vi "SelectChannels.vi"(6 "Controls Only?":bool, 8 "error in":errorcluster, 9 "Listbox Settings":T1, 10 "Previous Selection":T2[](array[typedef]), 11 "Root.BaseNodeType":refnum<k24>) -> (0 "error out":errorcluster, 1 "Listbox Settings Out":T1, 2 "Channel Selection":T2[](array[typedef]))   [LabVIEW 2012, in "TableSupportLib.lvlib"]
uses:
  TableSupportLib.lvlib
  NationalInstruments.VeriStand.SystemStorageUI
  Table_ChannelInfoCluster.ctl
  NationalInstruments.VeriStand.SystemStorage
  Table_ListboxSettings.ctl
  <vilib>/Utility/miscctls.llb/LVRowAndColumnTypeDef.ctl
  <vilib>/Utility/miscctls.llb/LVRowAndColumnUnsignedTypeDef.ctl
  <vilib>/NI Veristand/UI Controls/Tree and Alias Browser/Node Ref.ctl
  NationalInstruments.VeriStand
  <vilib>/NI/AMC/Read Termination Message.vi
  <vilib>/NI/AMC/Create Single Message.vi
  <vilib>/NI/AMC/Update Message Routing Info.vi
  Table_Globals.vi
  <vilib>/NI/AMC/Globals.vi
  <vilib>/NI/AMC/Send Message.vi
  NationalInstruments.VeriStand.SystemDefinitionAPI
  <vilib>/NI/AMC/AMC.lvlib
  <vilib>/NI Veristand/UI Controls/Tree and Alias Browser/NI_VS UI Tree Alias Browser.lvlib
panel:
  in  "Tab Control":enum32{"Channel Setup", "Listbox Setup"}(tab)
  in  "Select Channels":refnum<k24>(container)
  in  "Channels":i32[](listbox)
  in  "Remove":bool
  in  "Add":bool
  in  "Generate Template":bool
  in  "Path":path
  in  "Include Limits":bool
  in  "Poll Rate":u32(ring)=200 items=["15 Hz"=66, "10 Hz"=100, "5 Hz"=200, "1 Hz"=1000, ".5"=2000]
  in  "Bold":bool
  in  "Text Size":u32=13
  in  "Cancel":bool
  in  "OK":bool
  # "Rate"
  # "Limits"
  # "Text"
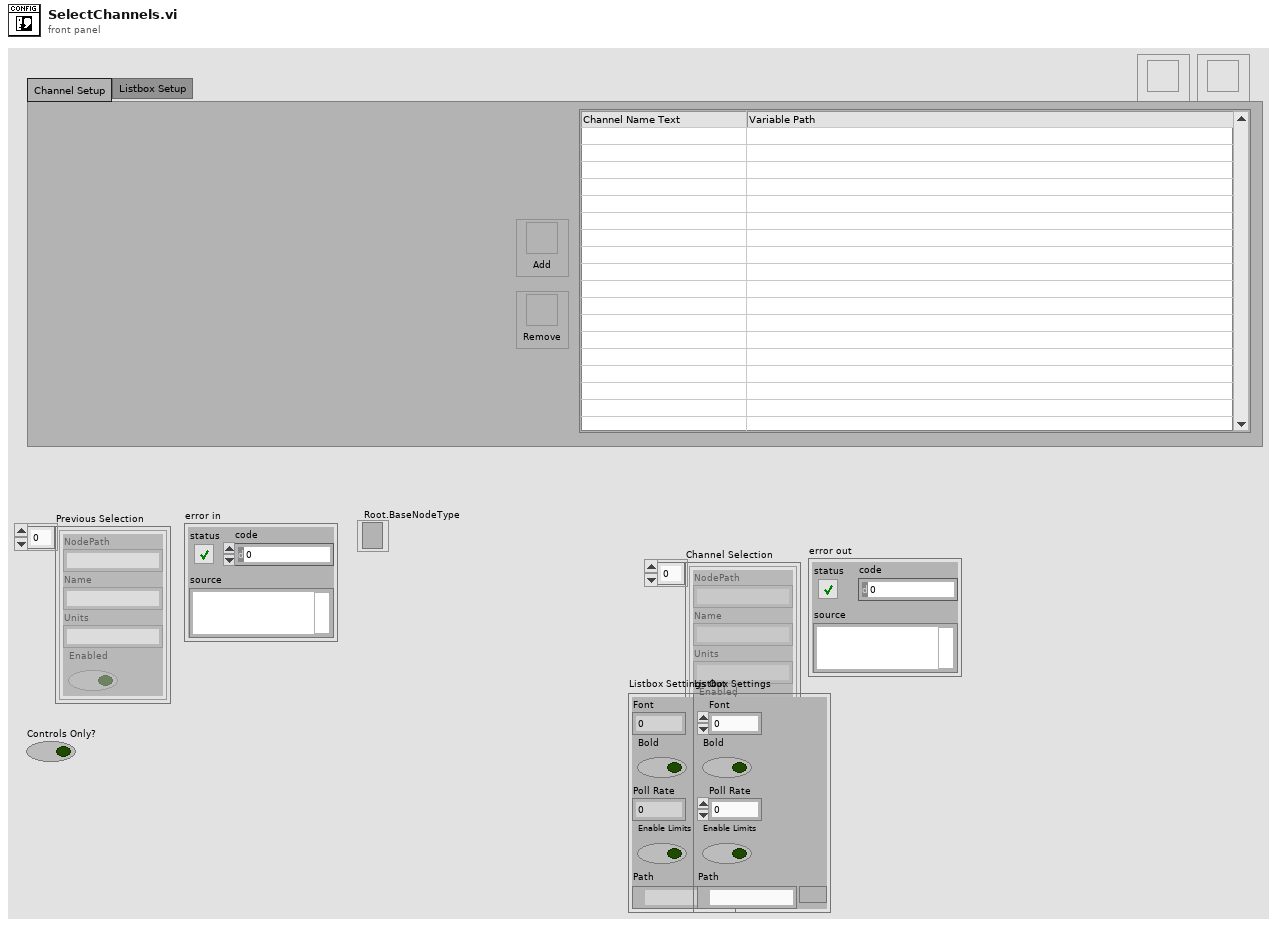
[diagram p1: front panel]
types:
  T1 = typedef "TableSupportLib.lvlib/Table_ListboxSettings.ctl" = cluster{"Font":u32, "Bold":bool, "Poll Rate":u32, "Enable Limits":bool, "Path":path}
  T2 = typedef "TableSupportLib.lvlib/Table_ChannelInfoCluster.ctl" = cluster{"NodePath":string, "Name":string, "Units":string, "Enabled":bool}
  T3 = typedef "NI_VS UI Tree Alias Browser.lvlib/Callback Type.ctl" = cluster{"Net Callbacks":refnum<k27>[], "Event":T4}
  T4 = typedef "NI_VS UI Tree Alias Browser.lvlib/Net Event Data Ref.ctl" = refnum<user-event>
  T5 = typedef "NI_VS UI Tree Alias Browser.lvlib/Tree Alias Browser Ref.ctl" = refnum<k24>
  T6 = typedef "AMC.lvlib/Message Queue.ctl" = refnum<queue>
  T7 = typedef "NI_VS UI Tree Alias Browser.lvlib/Node Ref.ctl" = refnum<k24>
  T8 = typedef "LVRowAndColumnUnsignedTypeDef.ctl" = cluster{"Row":u32, "Column":u32}
  T9 = typedef "LVRowAndColumnTypeDef.ctl" = cluster{"Row":i32, "Column":i32}
  T10 = enum16{"open", "replace", "create", "open or create", "replace or create", "replace or create with confirmation"}
  T11 = typedef "NI_VS UI Tree Alias Browser.lvlib/Net Event.ctl" = enum16{"SelectedItem", "DblClick"}
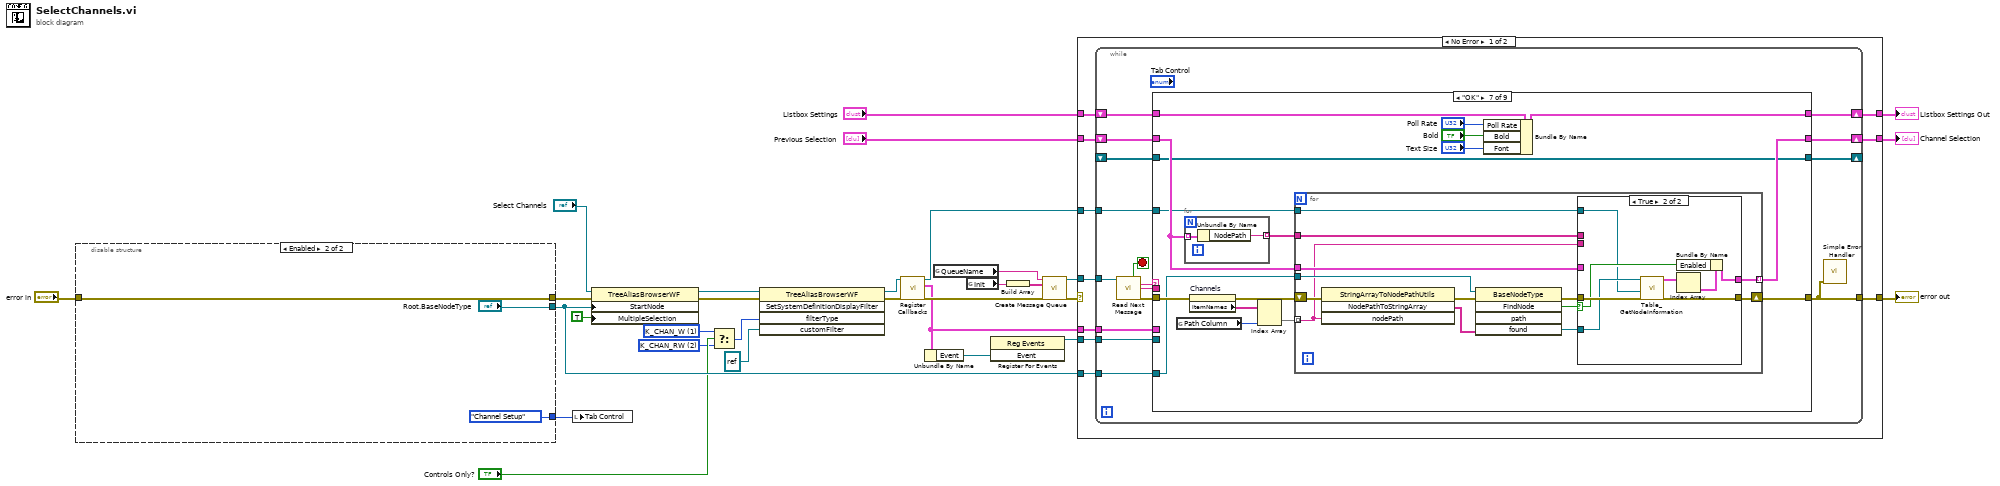
[diagram p0: block diagram]
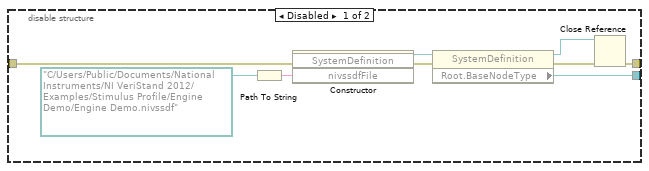
[diagram p2: hidden frame]
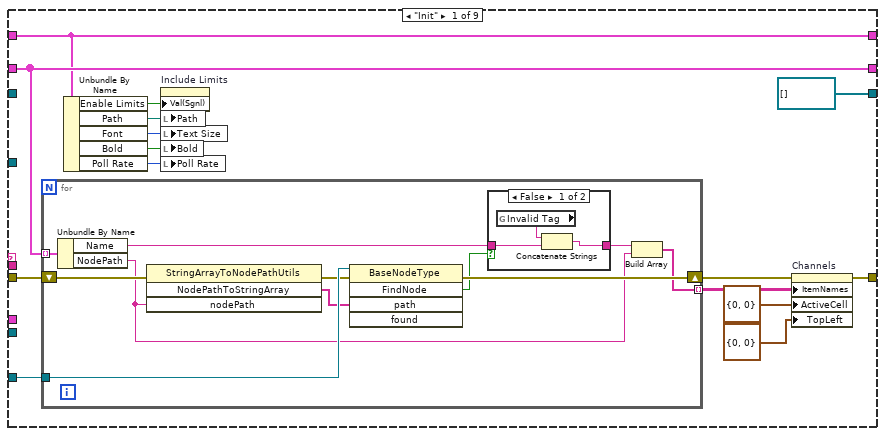
[diagram p3: hidden frame]
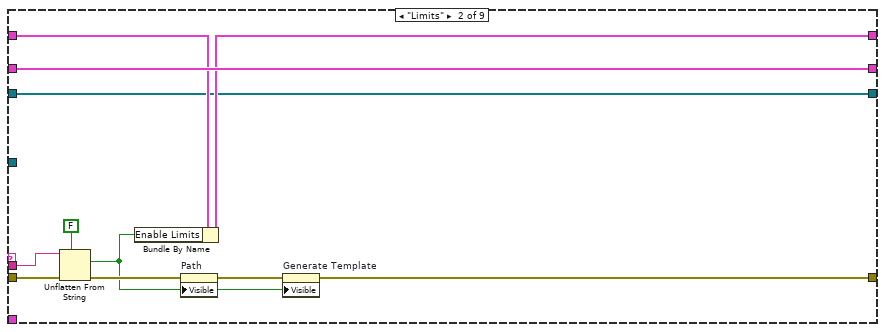
[diagram p5: hidden frame]
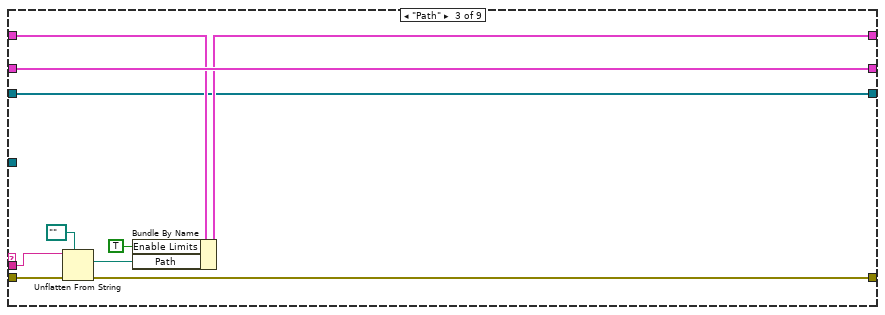
[diagram p6: hidden frame]
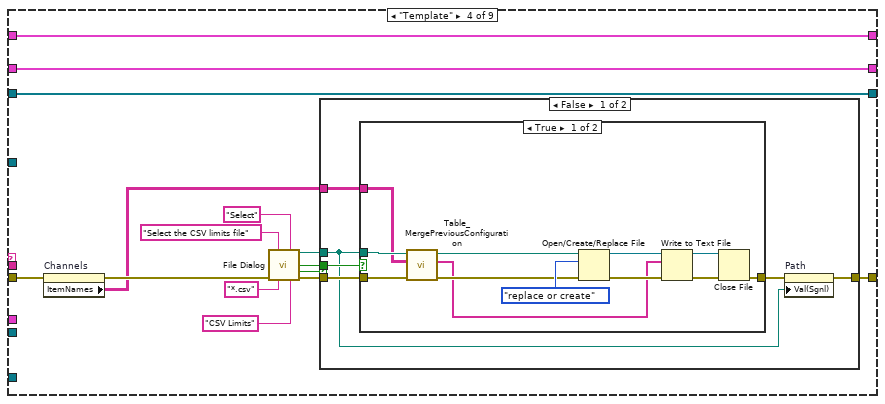
[diagram p7: hidden frame]
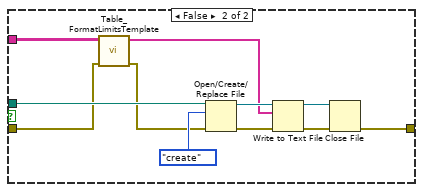
[diagram p8: hidden frame]
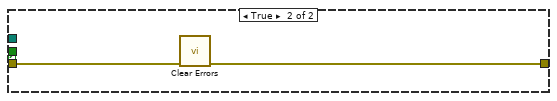
[diagram p9: hidden frame]
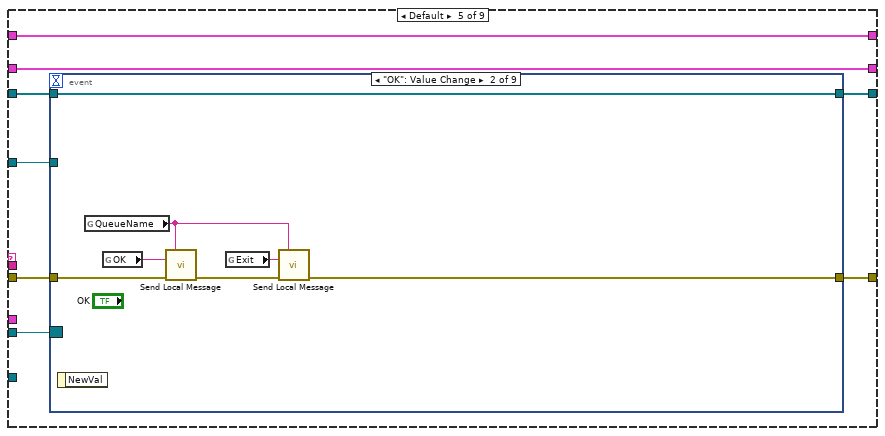
[diagram p10: hidden frame]
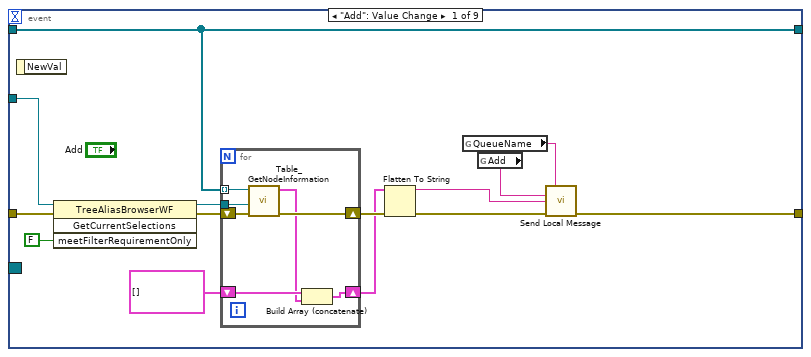
[diagram p11: hidden frame]
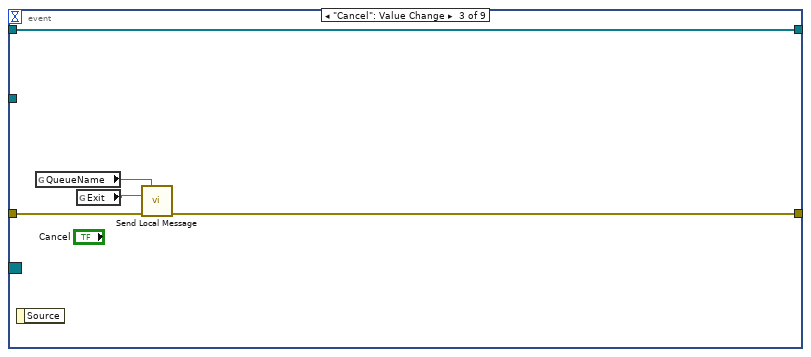
[diagram p12: hidden frame]
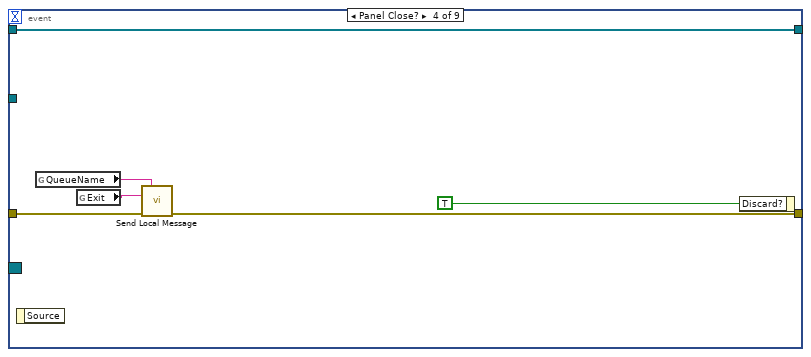
[diagram p13: hidden frame]
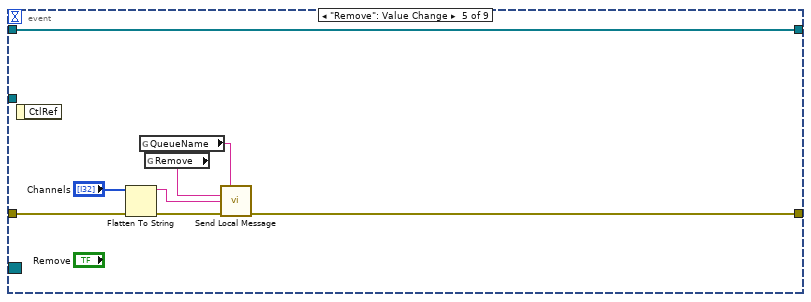
[diagram p14: hidden frame]
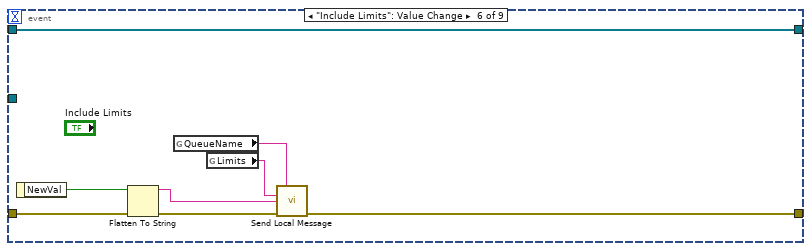
[diagram p15: hidden frame]
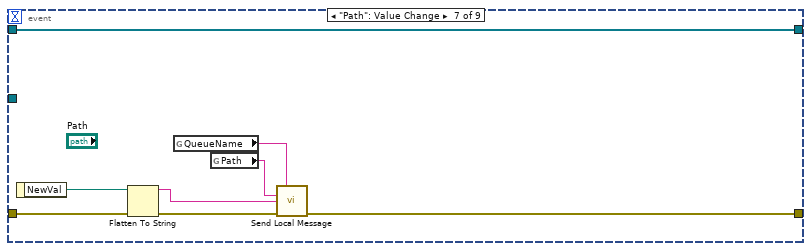
[diagram p16: hidden frame]
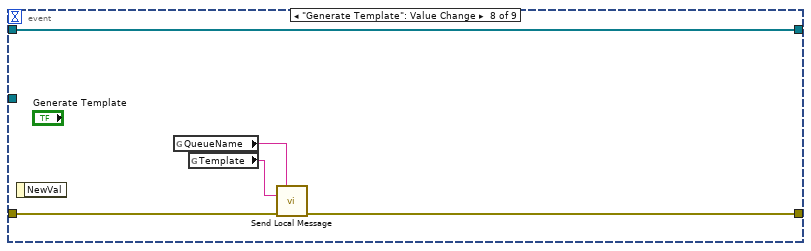
[diagram p17: hidden frame]
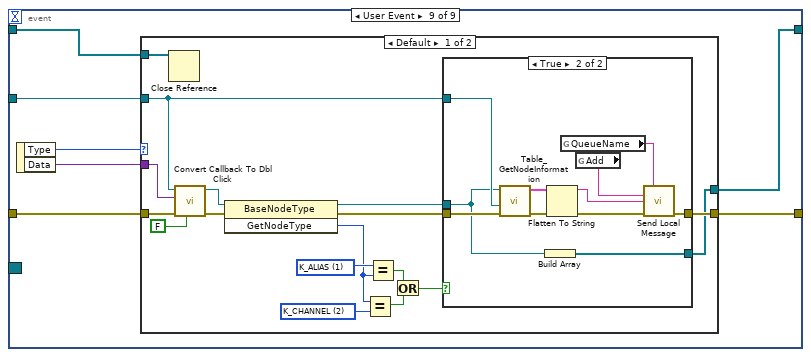
[diagram p18: hidden frame]
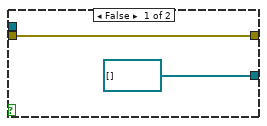
[diagram p19: hidden frame]
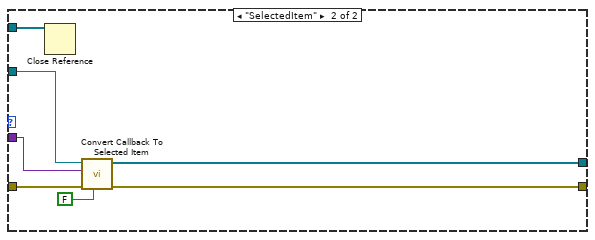
[diagram p20: hidden frame]
diagram:
  w9 = u8 1 items=["K_CHAN_R", "K_CHAN_W", "K_CHAN_RW", "K_CHAN_VOLT", "K_CHAN_FAULT", "K_ALL", "K_CUSTOM", "K_CHAN_R_VIS", "K_CHAN_W_VIS", "K_CHAN_RW_VIS", "K_CHAN_VOLT_VIS", "K_CHAN_FAULT_VIS", "K_WAVE", "K_WAVE_VIS", "K_WAVE_DBL", "K_WAVE_CDB", "K_WAVE_DBL_VIS", "K_WAVE_CDB_VIS"] ("filterType")
  w10 = u8 2 items=["K_CHAN_R", "K_CHAN_W", "K_CHAN_RW", "K_CHAN_VOLT", "K_CHAN_FAULT", "K_ALL", "K_CUSTOM", "K_CHAN_R_VIS", "K_CHAN_W_VIS", "K_CHAN_RW_VIS", "K_CHAN_VOLT_VIS", "K_CHAN_FAULT_VIS", "K_WAVE", "K_WAVE_VIS", "K_WAVE_DBL", "K_WAVE_CDB", "K_WAVE_DBL_VIS", "K_WAVE_CDB_VIS"] ("filterType")
  n1 = disable-structure shown="Enabled" {
    disable-tunnel: [w35 "Root.BaseNodeType"] -> w23
    disable-tunnel: [w32 w42] -> w19
    disable-tunnel: "error in" -> [w31 w42]
    disable-tunnel: [_ enum32{"Channel Setup", "Listbox Setup"}."Channel Setup" ("Tab Control")] -> w12
    frame Disabled {
      n2 = Path To String(path=path "C:/Users/Public/Documents/National Instruments/NI VeriStand 2012/Examples/Stimulus Profile/Engine Demo/Engine Demo.nivssdf") -> (string=w38:string)
      n3 = constructor class="SystemDefinition"(error in=w31, "nivssdfFile"=w38) -> (reference out=w37:refnum<k24>, error out=w36:errorcluster)  [unwired: 2 in, 2 out]
      n4 = property class="SystemDefinition"(reference=w37, error in=w36) -> (reference out=w34:refnum<k24>, error out=w33:errorcluster, "Root.BaseNodeType"=w35:refnum<k24>)
      n5 = Close Reference(reference=w34, error in (no error)=w33) -> (error out=w32:errorcluster)
    }
    frame Enabled {
    }
  }
  n6 = local write "Tab Control"(w12) -> ()
  n7 = property class="TreeAliasBrowserWF"(reference="Select Channels", error in=w19, "StartNode"=w23, "MultipleSelection"=TRUE) -> (reference out=w29:refnum<k24>, error out=w28:errorcluster)
  n8 = Select(t=w9, s="Controls Only?", f=w10) -> (s? t:f=w8:u8)
  n9 = invoke class="TreeAliasBrowserWF" method="SetSystemDefinitionDisplayFilter"(reference=w29, error in=w28, "filterType"=w8, "customFilter"=refnum<k24> refnum) -> (reference out=w5:refnum<k24>, error out=w7:errorcluster)  [unwired: 1 in, 3 out]
  n10 = call <vilib>:"Register Callbacks.vi"("error in (no error)"=w7, "Tree Alias"=w5) -> ("error out"=w6:errorcluster, "Callbacks"=w1:T3, "Tree Alias dup"=w4:T5)  [unwired: 7 in]
  n11 = Unbundle By Name(w1) -> ("Event"=w2:T4)
  n12 = global read "Table_Globals.vi" "QueueName"() -> (w25:string)
  n13 = global read "Table_Globals.vi" "Init"() -> (w21:string)
  n14 = register-events(w2) -> (reference out=w3:refnum<event-registration>)  [unwired: 2 in, 1 out]
  n15 = Build Array(w21) -> (w20:string[])
  n16 = call <vilib>:"Create Message Queue.vi"("message queue name"=w25, "initial message names"=w20, "error in"=w6) -> ("message queue out"=w26:T6, "error out"=w18:errorcluster)  [unwired: 11 in]
  n17 = case shown="No Error" w18 {
    selector: w18 -> [_ w401]
    tunnel: w4 -> [w52 _]
    tunnel: w26 -> [w51 _]
    tunnel: "Previous Selection" -> [w50 w402]
    tunnel: [w49 w400] -> w15
    tunnel: w23 -> [w48 _]
    tunnel: [w47 w402] -> w22
    tunnel: "Listbox Settings" -> [w46 w399]
    tunnel: [w45 w399] -> w13
    tunnel: w3 -> [w44 _]
    tunnel: w1 -> [w43 _]
    frame No Error {
      n18 = while {
        tunnel: w52 -> [w68]
        tunnel: w51 -> [w66]
        tunnel: [w59] -> w49
        tunnel: w48 -> [w62]
        shift-right: [w61] -> w47
        shift-left: w50 -> [w63]
        shift-right: [w57] -> w45
        shift-left: w46 -> [w58]
        tunnel: w44 -> [w56]
        shift-right: [w55] -> _
        shift-left: _ -> [w54]
        tunnel: w43 -> [w53]
        stop <- w60 stop-if-true
        n19 = call <vilib>:"Read Next Message.vi"("message queue in"=w66) -> ("exit process?"=w60:bool, "message name"=w65:string, "message value"=w64:string, "error out"=w67:errorcluster)  [unwired: 7 in, 4 out]
        n20 = case shown="\"OK\"" w65 {
          tunnel: w68 -> [_ _ _ _ w173 _ w318 w374 _]
          tunnel: w67 -> [w82 w108 w118 w132 w172 w298 w333 w368 w394]
          tunnel: [w79 w103 w117 w124 w171 w295 w329 w373 w383] -> w59
          tunnel: w64 -> [_ w107 w116 _ _ w297 _ _ w392]
          tunnel: w63 -> [w83 w109 w119 w134 w170 w296 w325 w377 w382]
          tunnel: w62 -> [w81 _ _ _ _ _ w331 _ _]
          tunnel: [w83 w109 w119 w134 w170 w296 w327 w377 w382] -> w61
          tunnel: [w72 w101 w112 w133 w169 w287 w319 w372 w379] -> w57
          tunnel: w58 -> [w72 w102 w113 w133 w169 w287 w320 w372 w379]
          tunnel: w56 -> [_ _ _ _ w168 _ _ w367 _]
          tunnel: [T7[] [] ("Selected Items") w99 w110 w120 w167 w286 w317 T7[] [] ("Selected Items") w378] -> w55
          tunnel: w54 -> [_ w99 w110 w120 w166 w286 w317 w371 w378]
          tunnel: w53 -> [_ _ _ _ _ _ _ w369 _]
          frame "Init" {
            n21 = for {
              tunnel: w81 -> [w94]
              shift-right: [w89] -> w80
              shift-left: w82 -> [w93]
              tunnel: w83 -> [w92] mode=indexing
              tunnel: [w87] -> w78 mode=indexing
              n22 = Unbundle By Name(w92) -> ("Name"=w86:string, "NodePath"=w84:string)
              n23 = invoke class="StringArrayToNodePathUtils" method="NodePathToStringArray"(error in=w93, "nodePath"=w84) -> (error out=w90:errorcluster, "NodePathToStringArray"=w91:string[])  [unwired: 2 in, 2 out]
              n24 = invoke class="BaseNodeType" method="FindNode"(reference=w94, error in=w90, "path"=w91) -> (error out=w89:errorcluster, "FindNode"=w88:bool)  [unwired: 2 in, 3 out]
              n25 = case shown="False" w88 {
                tunnel: w86 -> [w97 w98]
                tunnel: [w96 w98] -> w85
                frame False {
                  n26 = global read "Table_Globals.vi" "Invalid Tag"() -> (w95:string)
                  n27 = Concatenate Strings(w95, w97) -> (w96:string)
                }
                frame True {
                }
              }
              n28 = Build Array(w85, w84) -> (w87:string[])
            }
            n29 = Unbundle By Name(w72) -> ("Enable Limits"=w70:bool, "Path"=w71:path, "Font"=w73:u32, "Bold"=w74:bool, "Poll Rate"=w75:u32)
            n30 = property on="Include Limits" class="Bool (strict)"("Val(Sgnl)"=w70) -> ()  [unwired: 2 in, 2 out]
            n31 = local write "Path"(w71) -> ()
            n32 = local write "Text Size"(w73) -> ()
            n33 = local write "Bold"(w74) -> ()
            n34 = local write "Poll Rate"(w75) -> ()
            n35 = property on="Channels" class="MCListbox (strict)"(error in=w80, "ItemNames"=w78, "ActiveCell"=T9 {"Row"=0, "Column"=0} ("Active Cell:Active Cell"), "TopLeft"=T8 {"Row"=0, "Column"=0} ("Top Left Visible Cell")) -> (error out=w79:errorcluster)  [unwired: 1 in, 1 out]
          }
          frame "Limits" {
            n36 = Unflatten From String(type=FALSE, binary string=w107, error in (no error)=w108) -> (value=w100:bool, error out=w105:errorcluster)  [unwired: 2 in, 1 out]
            n37 = Bundle By Name(cluster=w102, "Enable Limits"=w100) -> (w101:T1)
            n38 = property on="Path" class="Path"(error in=w105, "Visible"=w100) -> (error out=w104:errorcluster)  [unwired: 1 in, 1 out]
            n39 = property on="Generate Template" class="Bool"(error in=w104, "Visible"=w100) -> (error out=w103:errorcluster)  [unwired: 1 in, 1 out]
          }
          frame "Path" {
            n40 = Unflatten From String(type=path "" ("Path"), binary string=w116, error in (no error)=w118) -> (value=w114:path, error out=w117:errorcluster)  [unwired: 2 in, 1 out]
            n41 = Bundle By Name(cluster=w113, "Enable Limits"=TRUE, "Path"=w114) -> (w112:T1)
          }
          frame "Template" {
            n42 = property on="Channels" class="MCListbox (strict)"(error in=w132) -> (error out=w131:errorcluster, "ItemNames"=w121:string[][])  [unwired: 1 in, 1 out]
            n43 = call "File Dialog"("prompt"="Select the CSV limits file" ("button label"), "button label"="Select", "error in"=w131, "pattern (all files)"="*.csv", "pattern label"="CSV Limits") -> ("selected path"=w123:path, "exists"=w122:bool, "cancelled"=w126:bool, "error out"=w125:errorcluster)  [unwired: 7 in]
            n44 = case shown="False" w126 {
              tunnel: w125 -> [w140 w165]
              tunnel: [w136 w164] -> w124
              tunnel: w123 -> [w135 _]
              tunnel: w122 -> [w139 _]
              tunnel: w121 -> [w138 _]
              frame False {
                n45 = case shown="True" w139 {
                  tunnel: w135 -> [w145 w163]
                  tunnel: [w148 w158] -> w137
                  tunnel: w140 -> [w146 w155]
                  tunnel: w138 -> [w144 w156]
                  frame True {
                    n46 = call "Table_MergePreviousConfiguration.vi"("error in (no error)"=w146, "Selections"=w144, "Path"=w145) -> ("error out"=w143:errorcluster, "Data"=w142:string[], "Path Out"=w141:path)  [unwired: 6 in]
                    n47 = Open/Create/Replace File(file path (use dialog)=w141, error in=w143, operation (0:open)=T10."replace or create") -> (refnum out=w152:refnum<file>, error out=w151:errorcluster)  [unwired: 3 in, 1 out]
                    n48 = Write to Text File(file (use dialog)=w152, text=w142, error in=w151) -> (refnum out=w149:refnum<file>, error out=w150:errorcluster)  [unwired: 1 in, 1 out]
                    n49 = Close File(refnum=w149, error in=w150) -> (error out=w148:errorcluster)  [unwired: 1 out]
                  }
                  frame False {
                    n50 = call "Table_FormatLimitsTemplate.vi"("error in (no error)"=w155, "Selections"=w156) -> ("error out"=w154:errorcluster, "Data"=w153:string[])  [unwired: 8 in]
                    n51 = Open/Create/Replace File(file path (use dialog)=w163, error in=w154, operation (0:open)=T10."create") -> (refnum out=w162:refnum<file>, error out=w161:errorcluster)  [unwired: 3 in, 1 out]
                    n52 = Write to Text File(file (use dialog)=w162, text=w153, error in=w161) -> (refnum out=w159:refnum<file>, error out=w160:errorcluster)  [unwired: 1 in, 1 out]
                    n53 = Close File(refnum=w159, error in=w160) -> (error out=w158:errorcluster)  [unwired: 1 out]
                  }
                }
                n54 = property on="Path" class="Path"(error in=w137, "Val(Sgnl)"=w135) -> (error out=w136:errorcluster)  [unwired: 1 in, 1 out]
              }
              frame True {
                n55 = call <vilib>:"Clear Errors.vi"("error in (no error)"=w165) -> ("error out"=w164:errorcluster)  [unwired: 6 in]
              }
            }
          }
          frame Default {
            n56 = event shown="[1] \"OK\": Value Change" {
              selector: w168 -> [_ _ _ _ _ _ _ _ _]
              dyn-events: _ -> [_ _ _ _ _ _ _ _ _]
              timeout: _ -> [_ _ _ _ _ _ _ _ _]
              tunnel: w172 -> [w185 w200 w205 w211 w216 w225 w233 w238 w247]
              tunnel: w173 -> [w186 _ _ _ _ _ _ _ w244]
              tunnel: [w180 w198 w203 w209 w215 w226 w234 w239 w246] -> w171
              tunnel: [w174 w195 w202 w207 w213 w221 w229 w237 w243] -> w167
              tunnel: w166 -> [w174 w195 w202 w207 w213 w221 w229 w237 w242]
              event "Add": Value Change {
                n57 = event-data() -> ()  [unwired: 1 in, 1 out]
                n58 = invoke class="TreeAliasBrowserWF" method="GetCurrentSelections"(reference=w186, error in=w185, "meetFilterRequirementOnly"=FALSE ("returnMeetFilterReqOnly")) -> (reference out=w176:T5, error out=w184:errorcluster)  [unwired: 1 in, 2 out]
                n59 = for {
                  shift-right: [w192] -> w178
                  shift-left: w184 -> [w194]
                  tunnel: w174 -> [w193] mode=indexing
                  shift-right: [w189] -> w175
                  shift-left: T2[] [] ("Channels") -> [w191]
                  tunnel: w176 -> [w188]
                  n60 = call "Table_GetNodeInformation.vi"("error in (no error)"=w194, "TreeBrowser"=w188, "reference"=w193) -> ("error IO"=w192:errorcluster, "Channels"=w190:T2[])  [unwired: 7 in]
                  n61 = Build Array (concatenate)(w191, w190) -> (w189:T2[])
                }
                n62 = Flatten To String(anything=w175, error in (no error)=w178) -> (data string=w182:string, error out=w183:errorcluster)  [unwired: 2 in, 1 out]
                n63 = global read "Table_Globals.vi" "QueueName"() -> (w179:string)
                n64 = global read "Table_Globals.vi" "Add"() -> (w181:string)
                n65 = call <vilib>:"Send Local Message.vi"("receiver process (\"\" - local)"=w179, "message name"=w181, "message value"=w182, "error in"=w183) -> ("error out"=w180:errorcluster)  [unwired: 9 in, 2 out]
              }
              event "OK": Value Change {
                n66 = event-data() -> ()  [unwired: 1 in, 1 out]
                n67 = global read "Table_Globals.vi" "QueueName"() -> (w197:string)
                n68 = global read "Table_Globals.vi" "OK"() -> (w201:string)
                n69 = call <vilib>:"Send Local Message.vi"("receiver process (\"\" - local)"=w197, "message name"=w201, "error in"=w200) -> ("error out"=w199:errorcluster)  [unwired: 10 in, 2 out]
                n70 = global read "Table_Globals.vi" "Exit"() -> (w196:string)
                n71 = call <vilib>:"Send Local Message.vi"("receiver process (\"\" - local)"=w197, "message name"=w196, "error in"=w199) -> ("error out"=w198:errorcluster)  [unwired: 10 in, 2 out]
              }
              event "Cancel": Value Change {
                n72 = event-data() -> ()  [unwired: 1 in, 1 out]
                n73 = global read "Table_Globals.vi" "QueueName"() -> (w204:string)
                n74 = global read "Table_Globals.vi" "Exit"() -> (w206:string)
                n75 = call <vilib>:"Send Local Message.vi"("receiver process (\"\" - local)"=w204, "message name"=w206, "error in"=w205) -> ("error out"=w203:errorcluster)  [unwired: 10 in, 2 out]
              }
              event Panel Close? {
                n76 = event-data() -> ()  [unwired: 1 in, 1 out]
                n77 = global read "Table_Globals.vi" "QueueName"() -> (w210:string)
                n78 = global read "Table_Globals.vi" "Exit"() -> (w212:string)
                n79 = call <vilib>:"Send Local Message.vi"("receiver process (\"\" - local)"=w210, "message name"=w212, "error in"=w211) -> ("error out"=w209:errorcluster)  [unwired: 10 in, 2 out]
                n80 = event-data("Discard?"=TRUE) -> ()  [unwired: 1 in, 1 out]
              }
              event "Remove": Value Change {
                n81 = event-data() -> ()  [unwired: 1 in, 1 out]
                n82 = Flatten To String(anything="Channels", error in (no error)=w216) -> (data string=w219:string, error out=w220:errorcluster)  [unwired: 2 in, 1 out]
                n83 = global read "Table_Globals.vi" "QueueName"() -> (w217:string)
                n84 = global read "Table_Globals.vi" "Remove"() -> (w218:string)
                n85 = call <vilib>:"Send Local Message.vi"("receiver process (\"\" - local)"=w217, "message name"=w218, "message value"=w219, "error in"=w220) -> ("error out"=w215:errorcluster)  [unwired: 9 in, 2 out]
              }
              event "Include Limits": Value Change {
                n86 = event-data() -> ("NewVal"=w223:bool)  [unwired: 1 in]
                n87 = Flatten To String(anything=w223, error in (no error)=w225) -> (data string=w222:string, error out=w224:errorcluster)  [unwired: 2 in, 1 out]
                n88 = global read "Table_Globals.vi" "QueueName"() -> (w227:string)
                n89 = global read "Table_Globals.vi" "Limits"() -> (w228:string)
                n90 = call <vilib>:"Send Local Message.vi"("receiver process (\"\" - local)"=w227, "message name"=w228, "message value"=w222, "error in"=w224) -> ("error out"=w226:errorcluster)  [unwired: 9 in, 2 out]
              }
              event "Path": Value Change {
                n91 = event-data() -> ("NewVal"=w231:path)  [unwired: 1 in]
                n92 = Flatten To String(anything=w231, error in (no error)=w233) -> (data string=w230:string, error out=w232:errorcluster)  [unwired: 2 in, 1 out]
                n93 = global read "Table_Globals.vi" "QueueName"() -> (w235:string)
                n94 = global read "Table_Globals.vi" "Path"() -> (w236:string)
                n95 = call <vilib>:"Send Local Message.vi"("receiver process (\"\" - local)"=w235, "message name"=w236, "message value"=w230, "error in"=w232) -> ("error out"=w234:errorcluster)  [unwired: 9 in, 2 out]
              }
              event "Generate Template": Value Change {
                n96 = event-data() -> ()  [unwired: 1 in, 1 out]
                n97 = global read "Table_Globals.vi" "QueueName"() -> (w240:string)
                n98 = global read "Table_Globals.vi" "Template"() -> (w241:string)
                n99 = call <vilib>:"Send Local Message.vi"("receiver process (\"\" - local)"=w240, "message name"=w241, "error in"=w238) -> ("error out"=w239:errorcluster)  [unwired: 10 in, 2 out]
              }
              event User Event {
                n100 = event-data() -> ("Type"=w248:T11, "Data"=w245:variant)  [unwired: 1 in]
                n101 = case shown="Default" w248 {
                  tunnel: w247 -> [w264 w285]
                  tunnel: [w253 w284] -> w246
                  tunnel: w245 -> [w265 w283]
                  tunnel: w244 -> [w256 w282]
                  tunnel: [w249 w281] -> w243
                  tunnel: w242 -> [w251 w280]
                  frame Default {
                    w263 = 2 items=["K_BASE", "K_ALIAS", "K_CHANNEL", "K_SECTION", "K_TARGET", "K_TARGETSECTION", "K_ROOT"] ("GetNodeType")
                    w262 = 1 items=["K_BASE", "K_ALIAS", "K_CHANNEL", "K_SECTION", "K_TARGET", "K_TARGETSECTION", "K_ROOT"] ("GetNodeType")
                    n102 = Close Reference(reference=w251) -> ()  [unwired: 1 in, 1 out]
                    n103 = call <vilib>:"Convert Callback To Dbl Click.vi"("Return Meet Filter Selection (T)"=FALSE, "error in"=w264, "Data"=w265, "TreeAliasBrowser Ref"=w256) -> ("error out"=w259:errorcluster, "Selected Node"=w258:T7)  [unwired: 5 in, 1 out]
                    n104 = invoke class="BaseNodeType" method="GetNodeType"(reference=w258, error in=w259) -> (reference out=w255:T7, error out=w254:errorcluster, "GetNodeType"=w257:i32)  [unwired: 1 in]
                    n105 = Equal?(x=w257, y=w263) -> (x = y?=w260:bool)
                    n106 = Equal?(x=w262, y=w257) -> (x = y?=w261:bool)
                    n107 = Or(x=w261, y=w260) -> (x .or. y?=w252:bool)
                    n108 = case shown="True" w252 {
                      tunnel: w256 -> [_ w278]
                      tunnel: w255 -> [_ w269]
                      tunnel: w254 -> [w267 w272]
                      tunnel: [w267 w271] -> w253
                      tunnel: [T7[] [] w268] -> w249
                      frame False {
                      }
                      frame True {
                        n109 = call "Table_GetNodeInformation.vi"("error in (no error)"=w272, "TreeBrowser"=w278, "reference"=w269) -> ("error IO"=w273:errorcluster, "Channels"=w270:T2[])  [unwired: 7 in]
                        n110 = Build Array(w269) -> (w268:T7[])
                        n111 = Flatten To String(anything=w270, error in (no error)=w273) -> (data string=w275:string, error out=w276:errorcluster)  [unwired: 2 in, 1 out]
                        n112 = global read "Table_Globals.vi" "QueueName"() -> (w277:string)
                        n113 = global read "Table_Globals.vi" "Add"() -> (w274:string)
                        n114 = call <vilib>:"Send Local Message.vi"("receiver process (\"\" - local)"=w277, "message name"=w274, "message value"=w275, "error in"=w276) -> ("error out"=w271:errorcluster)  [unwired: 9 in, 2 out]
                      }
                    }
                  }
                  frame "SelectedItem" {
                    n115 = Close Reference(reference=w280) -> ()  [unwired: 1 in, 1 out]
                    n116 = call <vilib>:"Convert Callback To Selected Item.vi"("Return Meet Filter Selection (T)"=FALSE, "error in"=w285, "Data"=w283, "TreeAliasBrowser Ref"=w282) -> ("error out"=w284:errorcluster, "Selected Items"=w281:T7[])  [unwired: 6 in]
                  }
                }
              }
            }
          }
          frame "Add" {
            n117 = Unflatten From String(type=w296, binary string=w297, error in (no error)=w298) -> (value=w292:T2[], error out=w294:errorcluster)  [unwired: 2 in, 1 out]
            n118 = global read "Table_Globals.vi" "Path Column"() -> (w288:i32)
            n119 = property on="Channels" class="MCListbox (strict)"(error in=w294) -> (error out=w293:errorcluster, "ItemNames"=w290:string[][])  [unwired: 1 in, 1 out]
            n120 = Index Array(array=w290, index (col)=w288) -> (element=w291:string[])  [unwired: 1 in]
            n121 = for {
              tunnel: w292 -> [w305] mode=indexing
              shift-right: [w299] -> w289
              shift-left: w290 -> [w302]
              tunnel: w291 -> [w303]
              n122 = Unbundle By Name(w305) -> ("Name"=w301:string, "NodePath"=w300:string)
              n123 = Search 1D Array(1D array=w303, element=w300) -> (index of element=w304:i32)  [unwired: 1 in]
              n124 = case shown="Default" w304 {
                selector: w304 -> [w310 _]
                tunnel: w302 -> [w311 w316]
                tunnel: w301 -> [w309 w315]
                tunnel: w300 -> [w308 w314]
                tunnel: [w306 w312] -> w299
                frame Default {
                  n125 = Build Array(w309, w308) -> (w307:string[])
                  n126 = Replace Array Subset(array=w311, new element=w307, index (row)=w310) -> (w306:string[][])  [unwired: 1 in]
                }
                frame -1 {
                  n127 = Build Array(w315, w314) -> (w313:string[])
                  n128 = Build Array (concatenate)(w316, w313) -> (w312:string[][])
                }
              }
            }
            n129 = property on="Channels" class="MCListbox (strict)"(error in=w293, "ItemNames"=w289) -> (error out=w295:errorcluster)  [unwired: 1 in, 1 out]
          }
          frame "OK" {
            n130 = global read "Table_Globals.vi" "Path Column"() -> (w332:i32)
            n131 = for {
              tunnel: w325 -> [w335] mode=indexing
              tunnel: [w334] -> w324 mode=indexing
              n132 = Unbundle By Name(w335) -> ("NodePath"=w334:string)
            }
            n133 = property on="Channels" class="MCListbox (strict)"(error in=w333) -> (error out=w330:errorcluster, "ItemNames"=w326:string[][])  [unwired: 1 in, 1 out]
            n134 = Index Array(array=w326, index (col)=w332) -> (element=w328:string[])  [unwired: 1 in]
            n135 = for {
              tunnel: w331 -> [w348]
              tunnel: w328 -> [w337] mode=indexing
              shift-right: [w346] -> w329
              shift-left: w330 -> [w347]
              tunnel: [w345] -> w327 mode=indexing
              tunnel: w325 -> [w339]
              tunnel: w324 -> [w338]
              tunnel: w318 -> [w336]
              n136 = invoke class="StringArrayToNodePathUtils" method="NodePathToStringArray"(error in=w347, "nodePath"=w337) -> (error out=w343:errorcluster, "NodePathToStringArray"=w344:string[])  [unwired: 2 in, 2 out]
              n137 = invoke class="BaseNodeType" method="FindNode"(reference=w348, error in=w343, "path"=w344) -> (error out=w342:errorcluster, "FindNode"=w340:bool, "found"=w341:refnum<k24>)  [unwired: 2 in, 2 out]
              n138 = case shown="True" w340 {
                selector: w340 -> [w354 w358]
                tunnel: [w353 w364] -> w346
                tunnel: [w355 w363] -> w345
                tunnel: w342 -> [w353 w362]
                tunnel: w341 -> [_ w360]
                tunnel: w339 -> [w356 _]
                tunnel: w338 -> [w352 _]
                tunnel: w337 -> [w351 _]
                tunnel: w336 -> [_ w357]
                frame False {
                  n139 = Search 1D Array(1D array=w352, element=w351) -> (index of element=w349:i32)  [unwired: 1 in]
                  n140 = Index Array(array=w356, index=w349) -> (element=w350:T2)
                  n141 = Bundle By Name(cluster=w350, "Enabled"=w354) -> (w355:T2)
                }
                frame True {
                  n142 = call "Table_GetNodeInformation.vi"("error in (no error)"=w362, "TreeBrowser"=w357, "reference"=w360) -> ("error IO"=w364:errorcluster, "Channels"=w361:T2[])  [unwired: 7 in]
                  n143 = Index Array(array=w361) -> (element=w359:T2)  [unwired: 1 in]
                  n144 = Bundle By Name(cluster=w359, "Enabled"=w358) -> (w363:T2)
                }
              }
            }
            n145 = Bundle By Name(cluster=w320, "Poll Rate"="Poll Rate", "Bold"="Bold", "Font"="Text Size") -> (w319:T1)
          }
          frame "Exit" {
            n146 = call <vilib>:"Unregister Callbacks.vi"("error in (no error)"=w368, "Callbacks"=w369) -> ("error out"=w366:errorcluster)  [unwired: 9 in]
            n147 = Unregister For Events(event registration refnum=w367, error in=w366) -> (error out=w365:errorcluster)
            n148 = invoke class="TreeAliasBrowserWF" method="ReleaseStartNode"(reference=w374, error in=w365) -> (reference out=w375:T5, error out=w376:errorcluster)  [unwired: 1 in, 1 out]
            n149 = Close Reference(reference=w371) -> ()  [unwired: 1 in, 1 out]
            n150 = Close Reference(reference=w375, error in (no error)=w376) -> (error out=w373:errorcluster)
          }
          frame "Remove" {
            n151 = local read "Channels"() -> (w393:i32[])
            n152 = Unflatten From String(type=w393, binary string=w392, error in (no error)=w394) -> (value=w389:i32[], error out=w391:errorcluster)  [unwired: 2 in, 1 out]
            n153 = property on="Channels" class="MCListbox (strict)"(error in=w391) -> (error out=w386:errorcluster, "ItemNames"=w390:string[][])  [unwired: 1 in, 1 out]
            n154 = call "Table_SortArrayFromHightoLow.vi"("Channels"=w389) -> ("Array"=w388:i32[])  [unwired: 10 in]
            n155 = for {
              tunnel: w388 -> [w397] mode=indexing
              shift-right: [w396] -> w387
              shift-left: w390 -> [w398]
              shift-right: [w395] -> w385
              shift-left: w386 -> [w395]
              n156 = Delete From Array(array=w398, index (row)=w397) -> (array with subset deleted=w396:string[][])  [unwired: 2 in, 1 out]
            }
            n157 = property on="Channels" class="MCListbox (strict)"(error in=w385, "ItemNames"=w387, "Value"=i32[] [] ("Channels"), "ActiveCell"=T9 {"Row"=0, "Column"=0} ("Active Cell:Active Cell"), "TopLeft"=T8 {"Row"=0, "Column"=0} ("Top Left Visible Cell")) -> (error out=w383:errorcluster)  [unwired: 1 in, 1 out]
          }
        }
        n158 = call <vilib>:"Simple Error Handler.vi"("error in (no error)"=w59) -> ()  [unwired: 4 in, 5 out]
      }
    }
    frame Error {
      n159 = call <vilib>:"Simple Error Handler.vi"("error in (no error)"=w401) -> ("error out"=w400:errorcluster)  [unwired: 4 in, 4 out]
    }
  }
  "error out" <- w15
  "Channel Selection" <- w22
  "Listbox Settings Out" <- w13
